vi "DVS_LabVIEWController_w_DAQ.vi"() -> ()   [LabVIEW 2013]
doc: "This example demonstrates temperature control and monitoring.\n\nNote:\nBefore start this VI is it necessary:\n\n- preconfigure some specific parameters that are not supported by this driver (e.g. PV-I/O Type, Linearization type, Alarm Input Values... ) by Quick Codes, or by Eurotherm iTools or by instrument front panel controls\n- enter correct VISA Resource Descriptor, Device Address and Baud Rate into front-panel controls"
uses:
  <vilib>/DAQmx/write.llb/DAQmx Write (Analog 1D DBL NChan 1Samp).vi
  <vilib>/DAQmx/read.llb/DAQmx Read (Analog 1D DBL NChan 1Samp).vi
  <vilib>/Utility/file.llb/Write To Spreadsheet File (string).vi
  <vilib>/Instr/_visa.llb/VISA Configure Serial Port (Instr).vi
  <vilib>/DAQmx/miscellaneous.llb/DAQmx Fill In Error Info.vi
  <instrlib>/Keithley 24XX/Public/Data/Read (Single Point).vi
  <instrlib>/Keithley 24XX/Keithley 24XX.lvlib
  <instrlib>/Eurotherm 32xx Series/Eurotherm 32xx Series.lvlib
panel:
  out "Waveform Chart 2":cluster{"f":dbl, "f":dbl}(graph)
  out "Waveform Chart 11":cluster{"Waveform":dbl, "Waveform":dbl}(graph)
  in  "Set vapor flow (sccm)":sgl min=0 max=200
  in  "Set gas flow (sccm)":sgl min=0 max=200
  out "Waveform Chart 10":dbl(graph)
  out "Vacuum Pressure (Torr)":dbl
  out "Waveform Chart 9":dbl(graph)
  out "Low pressure (Torr)":dbl
  out "Vapor flow (sccm)":dbl
  out "Gas flow (sccm)":dbl
  out "raw DVS DAQ data":dbl[](array[numeric])
  out "Waveform Chart 8":dbl(graph)
  out "High pressure (Torr)":dbl
  in  "Vacuum Data":bool
  in  "RapidOX":bool
  in  "Eurotherm Temp\nController":bool
  in  "4-wire?":bool
  in  "stop":bool
  in  "O2 PUMP":bool
  in  "QCM":bool
  in  "Keithley 2420":bool
  out "Data\nfile\npath":path
  in  "DATA COMMENTS":string
  out "ERRORS":errorcluster
  out "Starting time":string
  out "Elapsed (min)":dbl caption="Elapsed Time (s)"
  in  "Delay between data points (s)":dbl format="%#_13g"
  in  "Stop after (min)":dbl
  in  "Auto stop?":bool
  out "min remaining":dbl
  in  "Setpoint (C)":sgl=25.0
  out "Temp":T1(graph)
  out "Temp (C)":sgl
  in  "J-KEM":bool
  out "Freq (Hz)":dbl format="%.3e"
  out "R (Ohm)":dbl format="%.3e"
  out "Waveform Chart 7":T2(graph)
  out "Current Temp (C)":dbl
  in  "Setpoint (C)":dbl=25.0
  out "Current Setpoint (C)":dbl
  out "Waveform Chart 5":cluster{dbl, dbl}(graph)
  out "Waveform Chart":cluster{dbl}(graph)
  out "Torr":dbl
  out "%":dbl
  out "atm":dbl
  in  "Com Port":i32(ring) items=["Com 1", "Com 2", "Com 3", "Com 4", "Com 5", "Com 6", "COM 7", "COM 8", "COM 9", "COM 10", "COM 11", "COM 12", "com 13", "COM 14"]
  in  "Baud Rate 2":i32(ring)=2 items=["2400", "4800", "9600", "19200", "38400", "57600", "115200"]
  in  "Com Port 2":i32(ring) items=["Com 1", "Com 2", "Com 3", "Com 4", "Com 5", "Com 6", "COM 7", "COM 8", "COM 9", "COM 10", "COM 11", "COM 12", "com 13", "COM 14"]
  out "Waveform Chart 6":cluster{dbl}(graph)
  out "O2 Concentration (PPM)":dbl
  out "Resistance (Ohm)":sgl
  out "Waveform Chart 4":cluster{"Resistance":sgl}(graph)
  # "Keithley 2420\nRead Resistance"
  # "MKS Pressure Sensor"
  # "Configuring Instrument\n \nPlease Wait......\n\nChart will update in 20 sec"
  # "SRS QCM\nController"
  # "MKS Pressure Sensor"
  # "MKS Pressure Sensor"
  # "J-Kem Temp Control"
  # "O2 Partial Pressure"
  # "SetNag\nO2 Pump"
  # "Setup"
  # "Instruments Connected:"
  # "Timing"
  # "Eurotherm Temp Control"
  # "Rapidox O2\nSensor"
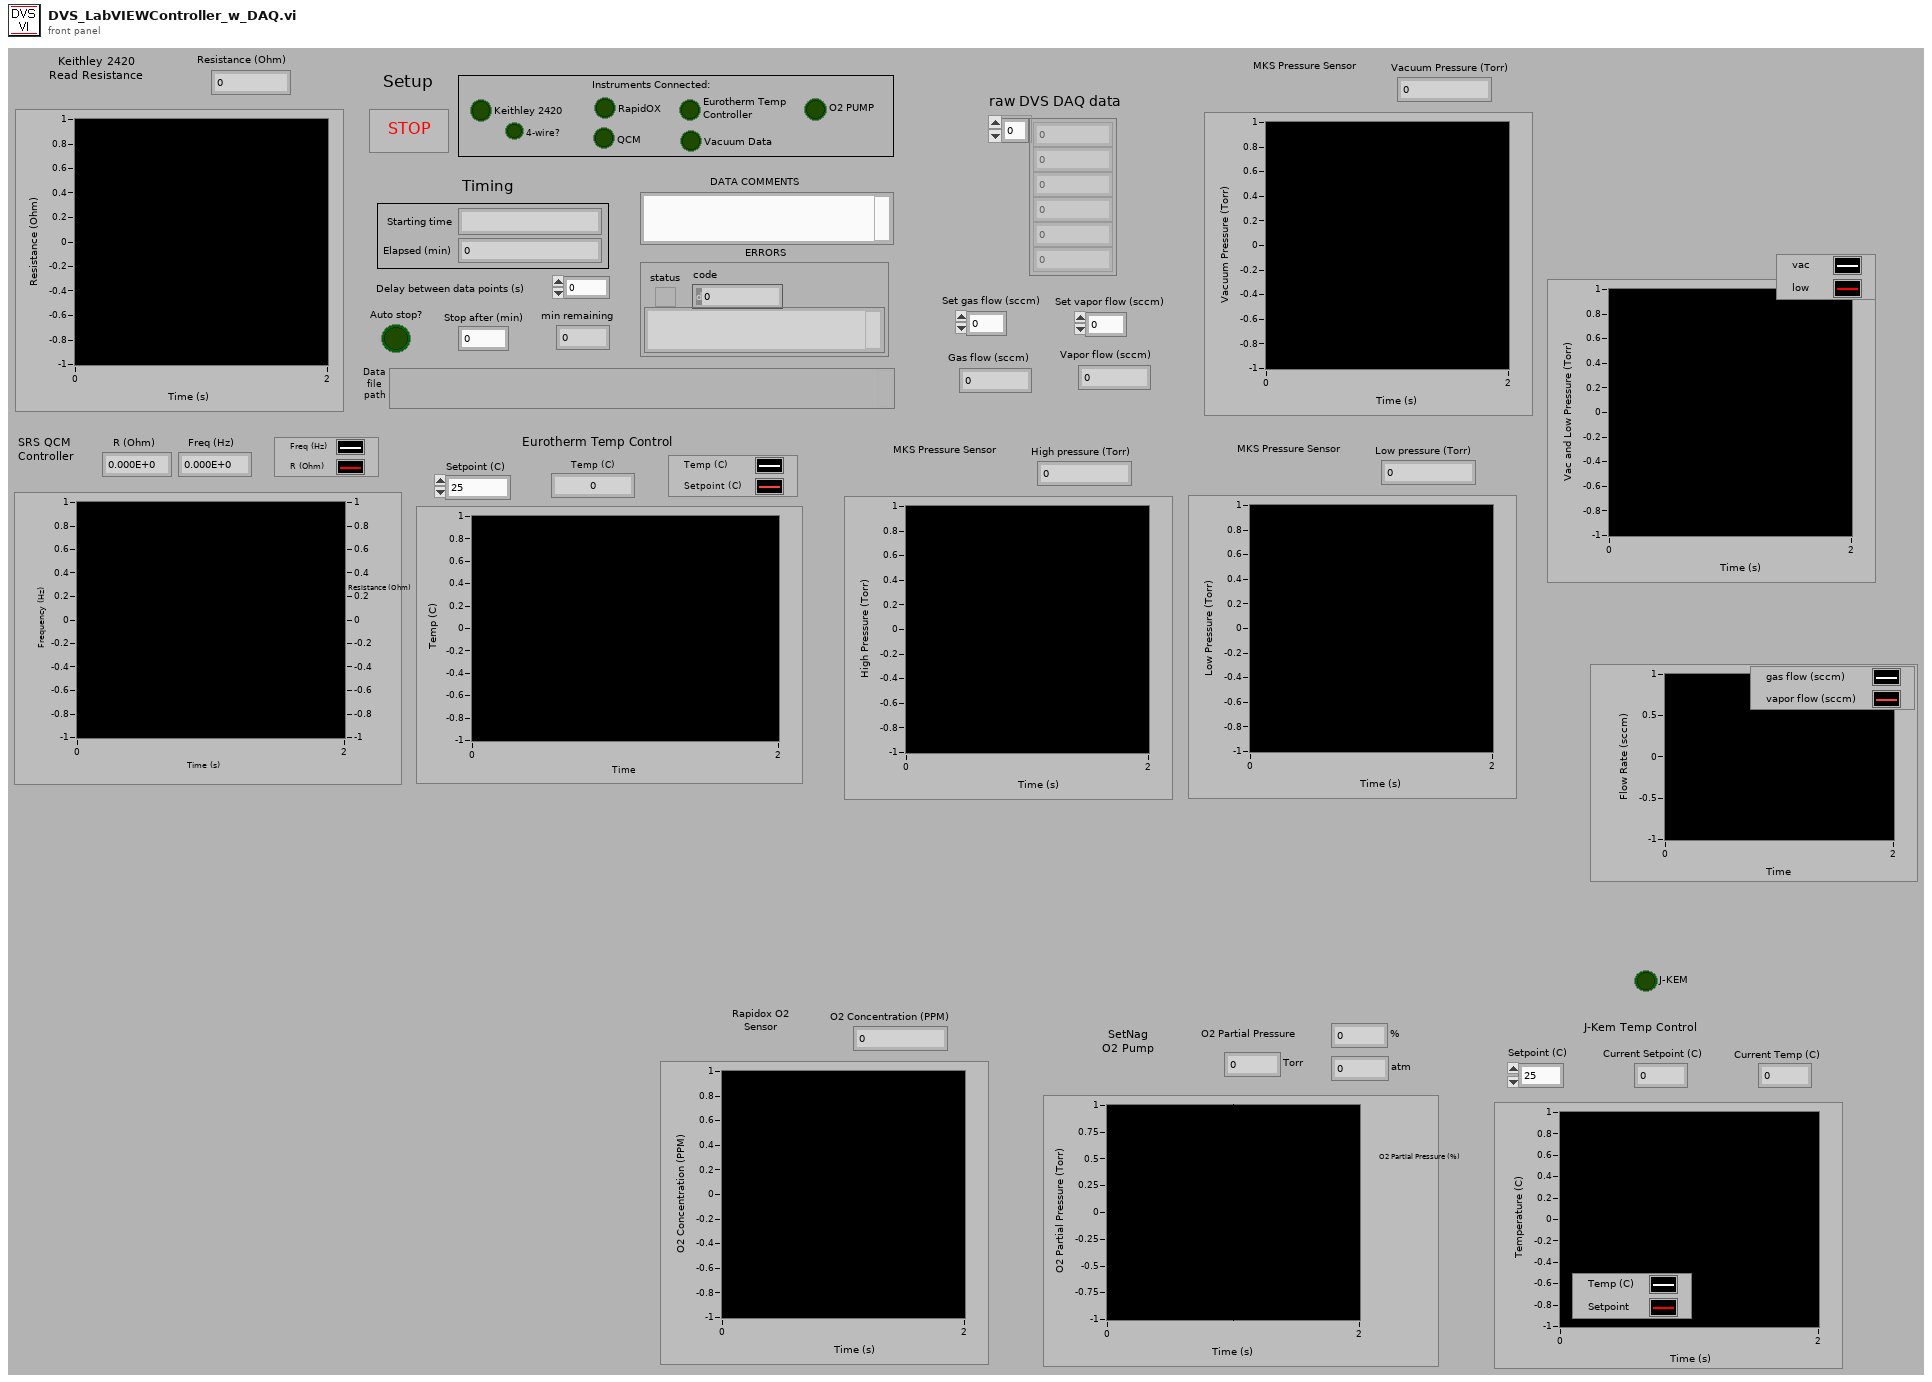
[diagram p1: front panel]
types:
  T1 = cluster{"Process Value":sgl, "Process Value":sgl}
  T2 = cluster{"Frequency out":dbl, "Resistance out":dbl}
  T3 = enum16{"open", "open or create", "create or replace", "create", "open (read only)"}
  T4 = cluster{bool, "Unit Address (1)":u8, "VISA resource name out":refnum<visa-resource-name>, "error out":errorcluster}
  T5 = cluster{"Process Value":sgl, "Setpoint Value 2":i16}[]
  T6 = cluster{"Baud Rate (19200)":u32, "Parity (0: None)":u16, "Break Length (0)":u16}
  T7 = enum16{"no parity", "odd parity", "even parity", "mark parity", "space parity"}
  T8 = cluster{bool, "VISA resource name":refnum<visa-resource-name>, "error out":errorcluster}
  T9 = cluster{bool, "VISA resource name out":refnum<visa-resource-name>, "error out":errorcluster}
  T10 = cluster{"Frequency out":dbl, "Resistance out":dbl}[]
  T11 = cluster{bool, "VISA out":refnum<visa-resource-name>, "error out":errorcluster}
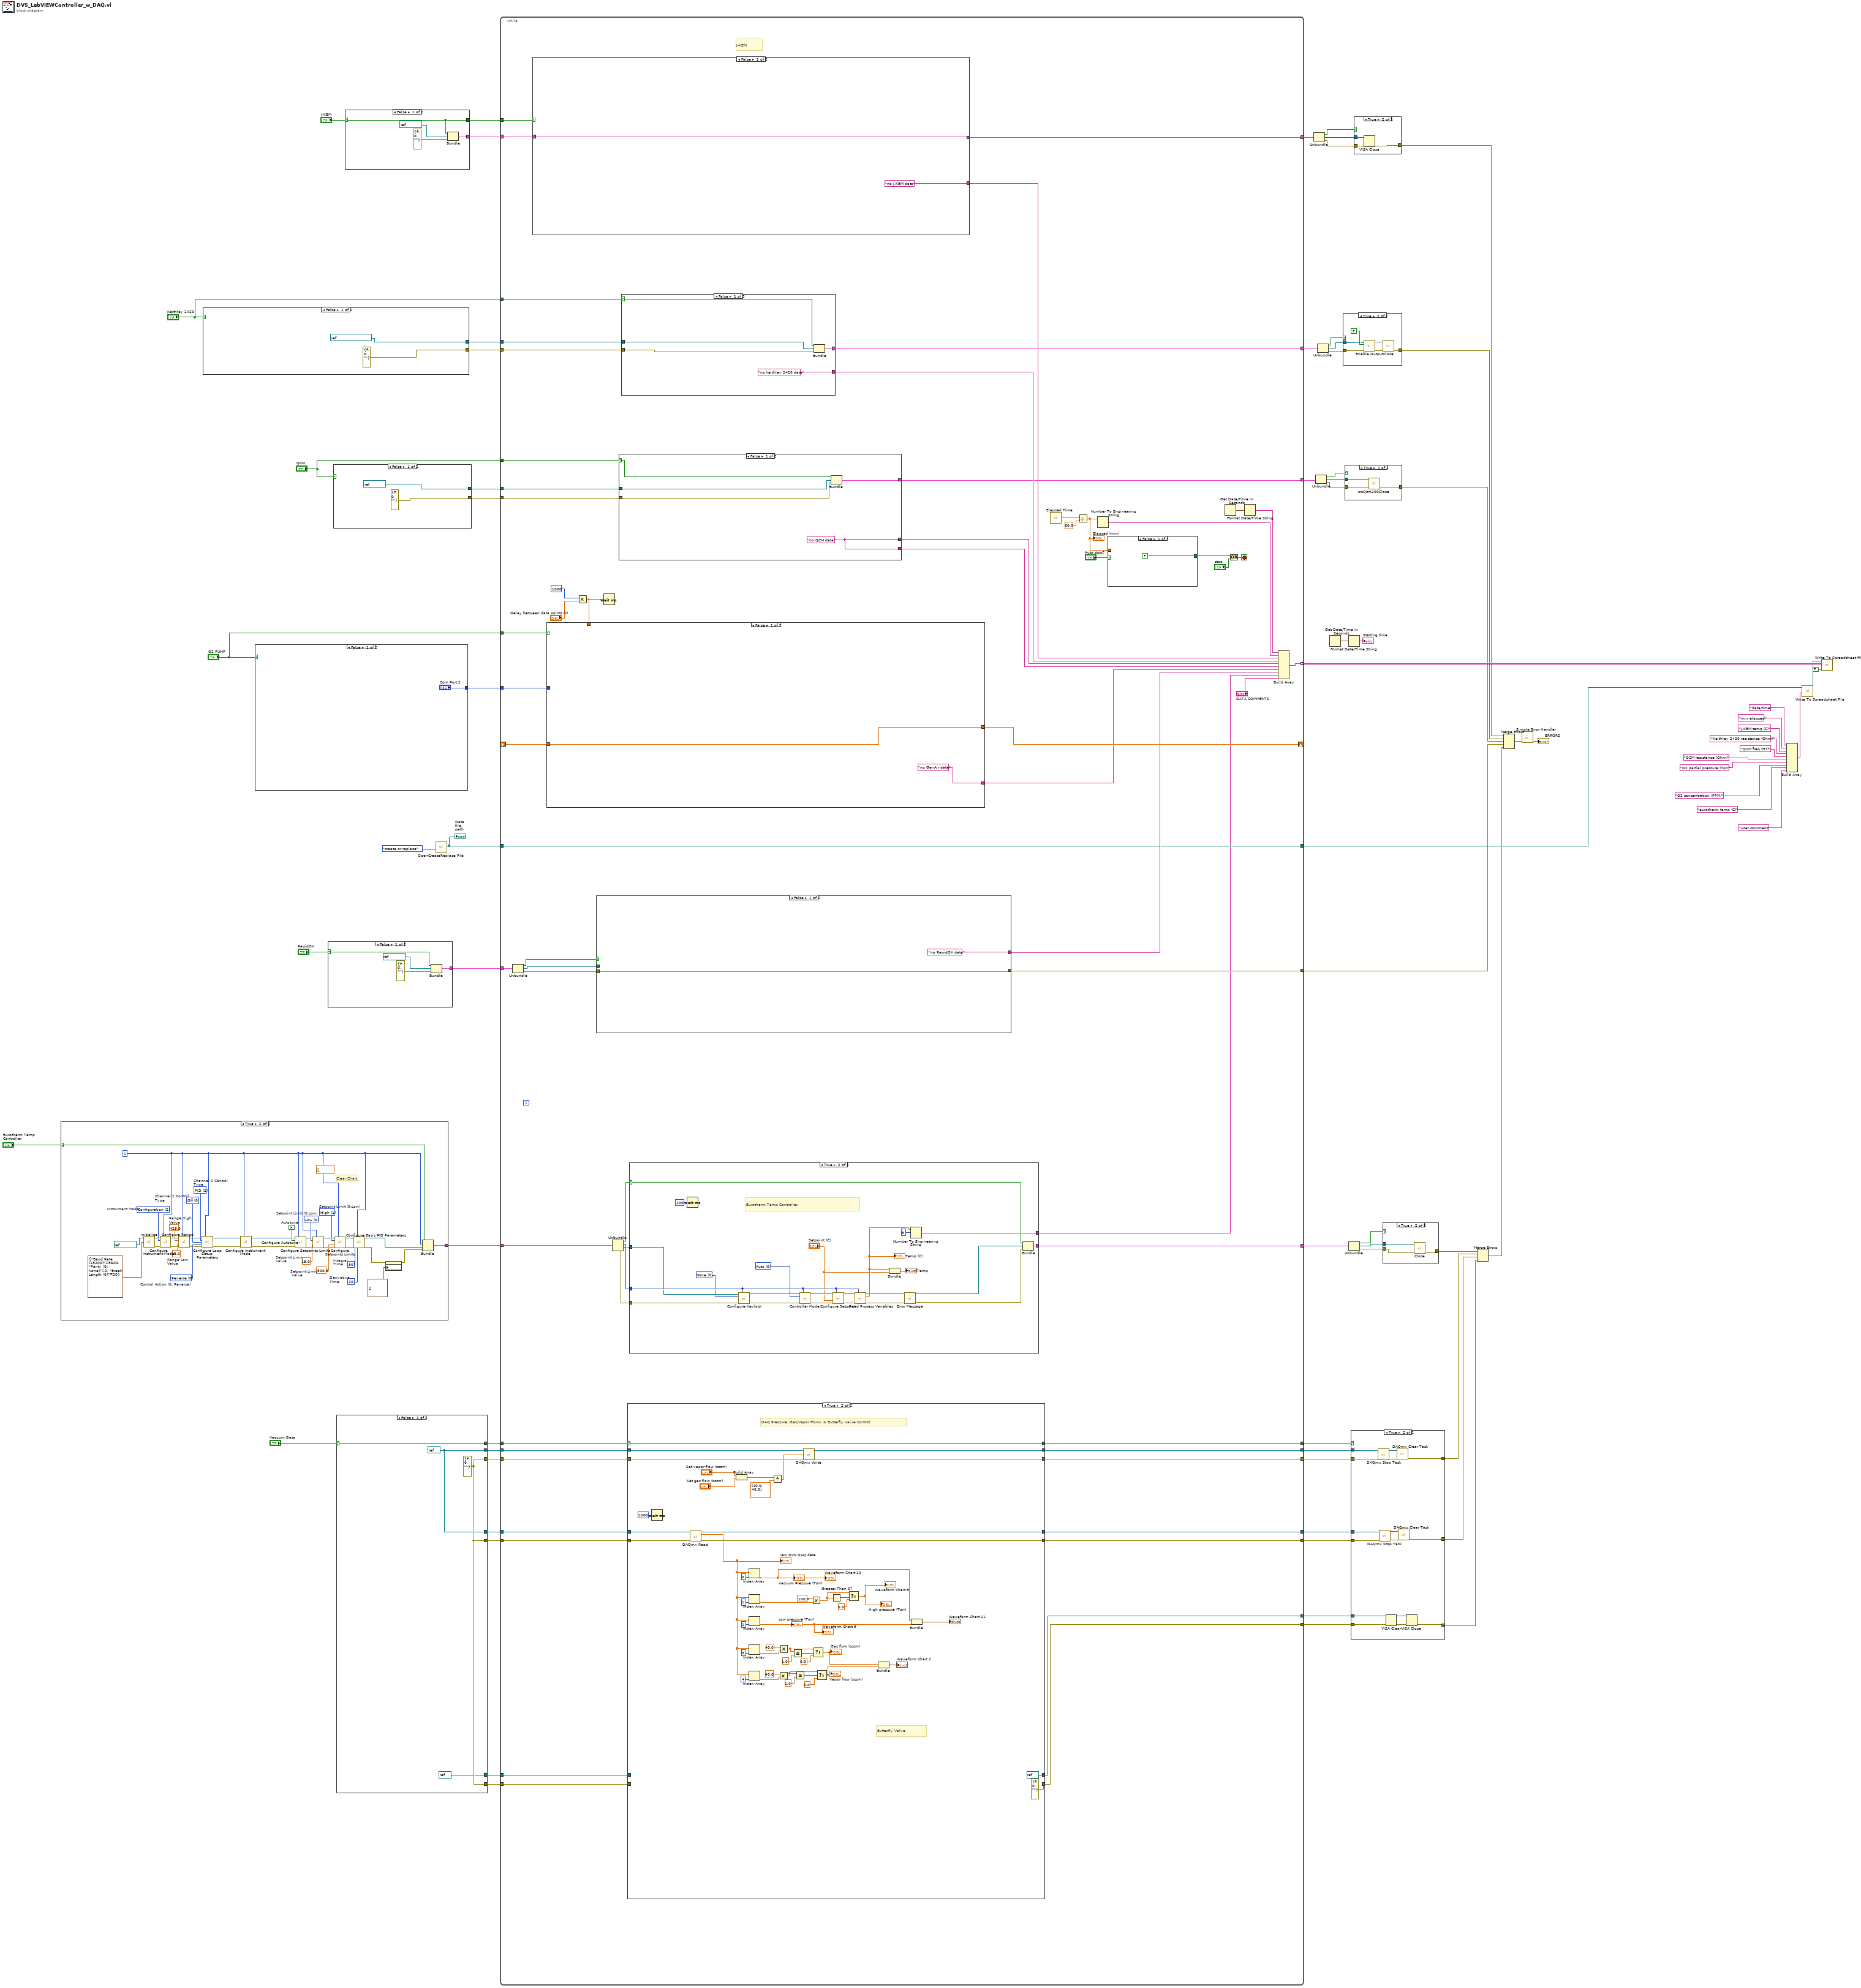
[diagram p0: block diagram]
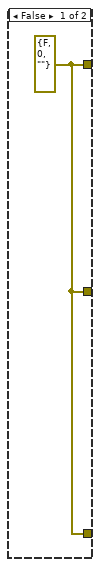
[diagram p2: hidden frame]
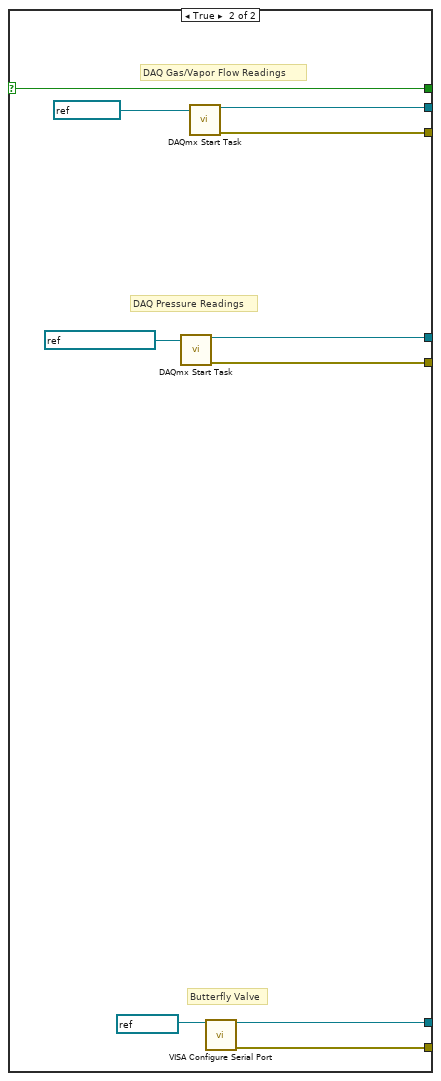
[diagram p3: hidden frame]
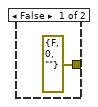
[diagram p4: hidden frame]
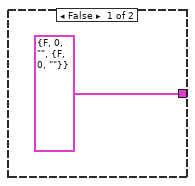
[diagram p5: hidden frame]
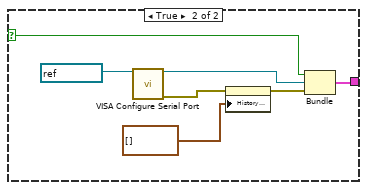
[diagram p6: hidden frame]
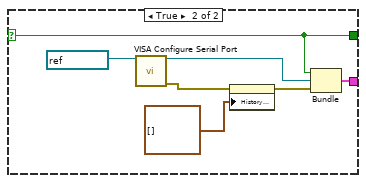
[diagram p8: hidden frame]
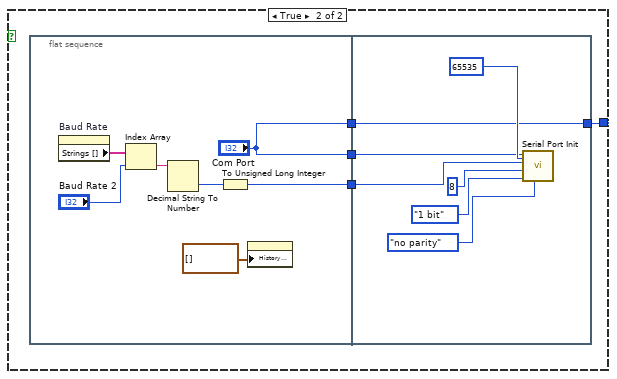
[diagram p9: hidden frame]
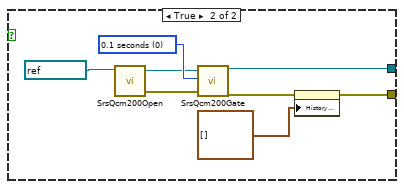
[diagram p11: hidden frame]
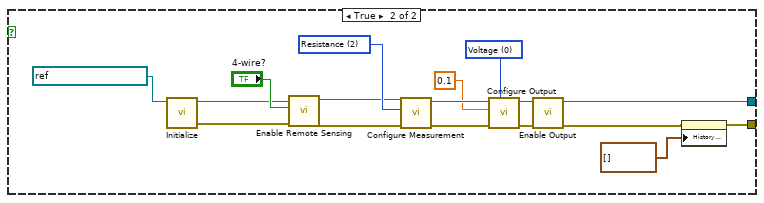
[diagram p13: hidden frame]
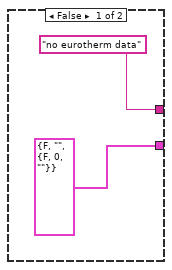
[diagram p15: hidden frame]
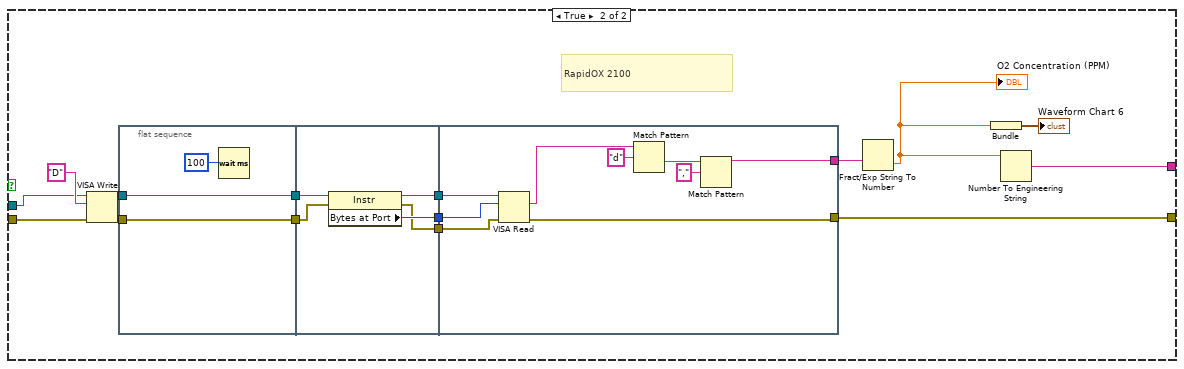
[diagram p16: hidden frame]
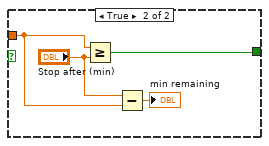
[diagram p17: hidden frame]
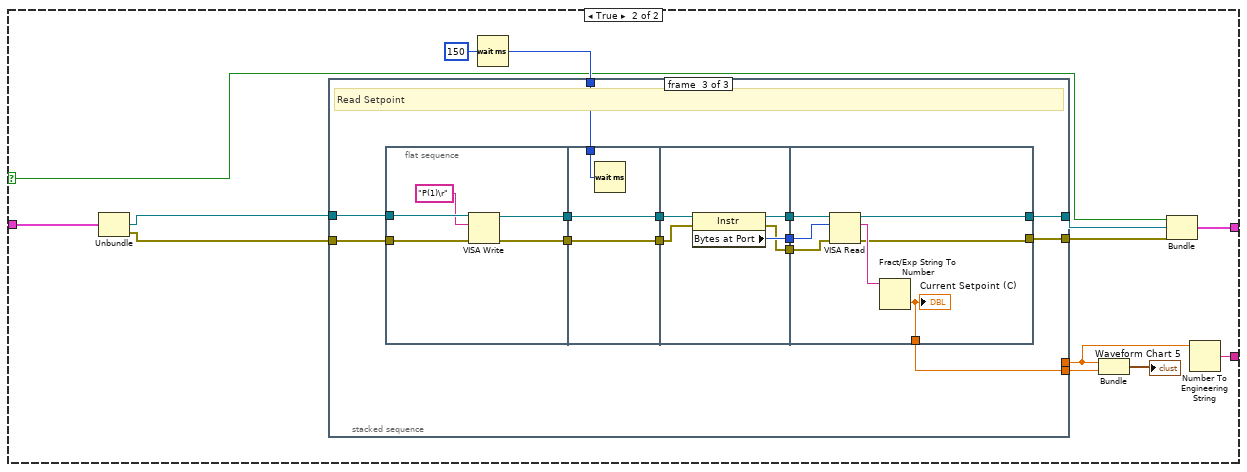
[diagram p18: hidden frame]
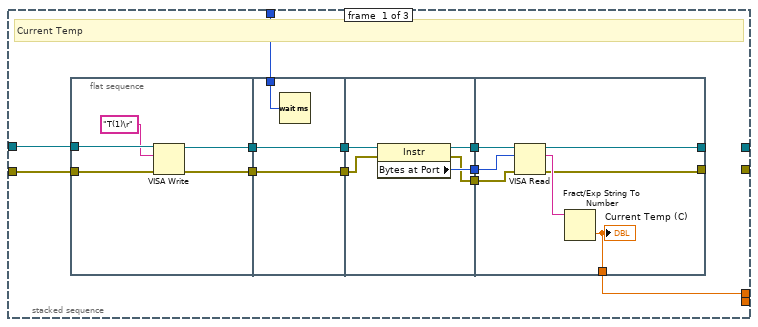
[diagram p19: hidden frame]
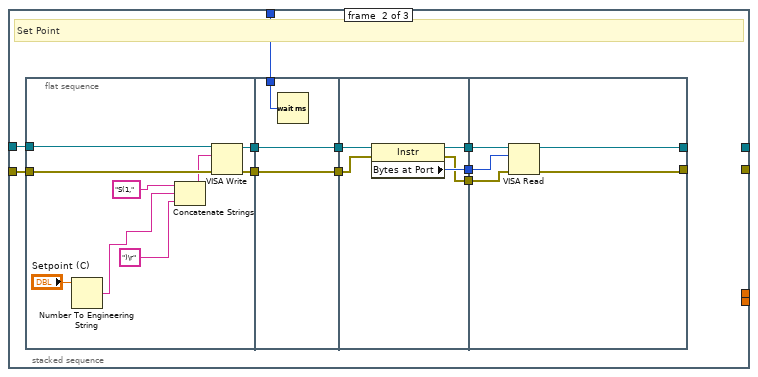
[diagram p20: hidden frame]
diagram:
  n1 = case shown="True" "Eurotherm Temp\nController" {
    selector: "Eurotherm Temp\nController" -> [_ w88]
    tunnel: [T4 {FALSE, "Unit Address (1)"=0, "VISA resource name out"="", "error out"={"status"=FALSE, "code"=0, "source"=""}} w85] -> w26
    frame False {
    }
    frame True {
      w87 = u8 1 ("Unit Address (1)")
      (unwired) sgl[] [] ("History Data")
      w92 = sgl 500.0  # Setpoint Limit  Value
      w95 = sgl 15.0  # Range Low  Value
      w96 = sgl 425.0  # Range High Value
      w97 = u16 0 items=["Reverse", "Direct"]  # Control Action (0: Reverse)
      w98 = u16 0 items=["Low", "High"]  # Setpoint Limit (0:Low)
      w99 = u16 1 items=["Low", "High"]  # Setpoint Limit (0:Low)
      w100 = 10  # Derivative  Time
      w101 = 50  # Integral  Time
      w102 = sgl 15.0  # Setpoint Limit  Value
      w107 = FALSE  # Autotune
      w110 = u8 0 items=["Off", "On/Off", "PID", "VPU", "VPB"]  # Channel 2 Control  Type
      w111 = u8 2 items=["Off", "On/Off", "PID", "VPU", "VPB"]  # Channel 1 Control  Type
      w114 = u8 2 items=["Normal", "StandBy", "Configuration"]  # Instrument Mode
      # "Clear Chart"
      n2 = call <instrlib>:"Initialize.vi"("VISA resource name"=refnum<visa-resource-name> "COM4", "Serial Configuration"=T6 {"Baud Rate (19200)"=9600, "Parity (0: None)"=0, "Break Length (0)"=20}) -> ("VISA resource name out"=w115:refnum<visa-resource-name>, "error out"=w91:errorcluster)  [unwired: 12 in]
      n3 = call <instrlib>:"Configure Instrument Mode.vi"("VISA resource name"=w115, "Unit Address (1)"=w87, "Instrument Mode (0: Normal)"=w114, "error in (no error)"=w91) -> ("VISA resource name out"=w113:refnum<visa-resource-name>, "error out"=w112:errorcluster)  [unwired: 10 in]
      n4 = call <instrlib>:"Configure Range.vi"("VISA resource name"=w113, "Unit Address (1)"=w87, "Range High (0)"=w96, "Range Low (0)"=w95, "error in (no error)"=w112) -> ("VISA resource name out"=w94:refnum<visa-resource-name>, "error out"=w93:errorcluster)  [unwired: 9 in]
      n5 = call <instrlib>:"Configure Loop Setup Parameters.vi"("VISA resource name"=w94, "Unit Address (1)"=w87, "Channel 1 Control Algorithm (0: Off)"=w111, "Channel 2 Control Algorithm (0: Off)"=w110, "Control Action (0: Reverse)"=w97, "error in (no error)"=w93) -> ("VISA resource name out"=w80:refnum<visa-resource-name>, "error out"=w81:errorcluster)  [unwired: 8 in]
      n6 = call <instrlib>:"Configure Instrument Mode.vi"("VISA resource name"=w80, "Unit Address (1)"=w87, "error in (no error)"=w81) -> ("VISA resource name out"=w79:refnum<visa-resource-name>, "error out"=w78:errorcluster)  [unwired: 11 in]
      n7 = call <instrlib>:"Configure Autotune.vi"("VISA resource name"=w79, "Unit Address (1)"=w87, "Enable Autotune  (False: Disable)"=w107, "error in (no error)"=w78) -> ("VISA resource name out"=w106:refnum<visa-resource-name>, "error out"=w105:errorcluster)  [unwired: 10 in]
      n8 = call <instrlib>:"Configure Setpoints Limits.vi"("VISA resource name"=w106, "Unit Address (1)"=w87, "Setpoint Limit (0:Low)"=w98, "Setpoint Limit Value (0)"=w102, "error in (no error)"=w105) -> ("VISA resource name out"=w109:refnum<visa-resource-name>, "error out"=w108:errorcluster)  [unwired: 9 in]
      n9 = call <instrlib>:"Configure Setpoints Limits.vi"("VISA resource name"=w109, "Unit Address (1)"=w87, "Setpoint Limit (0:Low)"=w99, "Setpoint Limit Value (0)"=w92, "error in (no error)"=w108) -> ("VISA resource name out"=w104:refnum<visa-resource-name>, "error out"=w103:errorcluster)  [unwired: 9 in]
      n10 = call <instrlib>:"Configure Basic PID Parameters.vi"("VISA resource name"=w104, "Unit Address (1)"=w87, "Integral Time (1)"=w101, "error in (no error)"=w103, "Derivative Time (0)"=w100) -> ("VISA resource name out"=w86:refnum<visa-resource-name>, "error out"=w83:errorcluster)  [unwired: 9 in]
      n11 = property on="Temp" class="WFChart (strict)"(error in=w83, "History Data"=T5 []) -> (error out=w82:errorcluster)  [unwired: 1 in, 1 out]
      n12 = Bundle(w88, "Unit Address (1)"=w87, "VISA resource name out"=w86, "error out"=w82) -> (w85:T4)  [unwired: 1 in]
    }
  }
  n13 = case shown="False" "Keithley 2420" {
    tunnel: [refnum<visa-resource-name> "GPIB1::24::INSTR" ("VISA resource name") w122] -> w70
    tunnel: [errorcluster {"status"=FALSE, "code"=0, "source"=""} ("error out") w125] -> w69
    frame False {
    }
    frame True {
      w128 = u16 0 items=["Voltage", "Current"] ("Source Mode  (0: Voltage)")
      w133 = u16 2 items=["Volts", "Current", "Resistance"] ("Function (0: Volts)")
      n14 = call <instrlib>:"Initialize.vi"("VISA resource name"=refnum<visa-resource-name> "GPIB1::24::INSTR") -> ("error out"=w118:errorcluster, "VISA resource name out"=w121:refnum<visa-resource-name>)  [unwired: 9 in]
      n15 = call <instrlib>:"Enable Remote Sensing.vi"("error in (no error)"=w118, "Enable Remote Sensing (T: Enable)"="4-wire?", "VISA resource name"=w121) -> ("error out"=w119:errorcluster, "VISA resource name out"=w120:refnum<visa-resource-name>)  [unwired: 7 in]
      n16 = call <instrlib>:"Configure Measurement.vi"("error in (no error)"=w119, "Function (0: Volts)"=w133, "VISA resource name"=w120) -> ("error out"=w132:errorcluster, "VISA resource name out"=w131:refnum<visa-resource-name>)  [unwired: 7 in]
      n17 = call <instrlib>:"Configure Output.vi"("Source Mode  (0: Voltage)"=w128, "error in (no error)"=w132, "Output Level (0)"=0.1 ("Output Level (V)"), "VISA resource name"=w131) -> ("error out"=w130:errorcluster, "VISA resource name out"=w129:refnum<visa-resource-name>)  [unwired: 6 in]
      n18 = call <instrlib>:"Enable Output.vi"("error in (no error)"=w130, "VISA resource name"=w129) -> ("error out"=w123:errorcluster, "VISA resource name out"=w122:refnum<visa-resource-name>)  [unwired: 8 in]
      n19 = property on="Waveform Chart 4" class="WFChart (strict)"(error in=w123, "History Data"=cluster{"Resistance":sgl}[] []) -> (error out=w125:errorcluster)  [unwired: 1 in, 1 out]
    }
  }
  n20 = case shown="False" "O2 PUMP" {
    tunnel: ["Com Port 2" w136] -> w64
    frame False {
    }
    frame True {
      n21 = flat-sequence {
        tunnel: ["Com Port"] -> w139
        tunnel: [w142] -> w138
        tunnel: ["Com Port"] -> w137
        tunnel: w139 -> [w148]
        tunnel: w138 -> [w147]
        tunnel: w137 -> [w149]
        tunnel: [w149] -> w136
        frame #0 {
          n22 = property on="Baud Rate" class="Ring (strict)"() -> ("Strings []"=w144:string[])  [unwired: 2 in, 2 out]
          n23 = Index Array(array=w144, index="Baud Rate 2") -> (element=w145:string)
          n24 = Decimal String To Number(string=w145) -> (number=w143:i32)  [unwired: 2 in, 1 out]
          n25 = To Unsigned Long Integer(number=w143) -> (unsigned 32bit integer=w142:u32)
          n26 = property on="Waveform Chart" class="WFChart (strict)"("History Data"=cluster{dbl}[] []) -> ()  [unwired: 2 in, 2 out]
        }
        frame #1 {
          n27 = call <vilib>:"Serial Port Init.vi"("parity"=T7."no parity", "buffer size"=u16 65535, "stop bits"=enum16{"1 bit", "1.5 bits", "2 bits"}."1 bit", "data bits"=u16 8, "baud rate"=w147, "port number"=w148) -> ()  [unwired: 1 in, 1 out]
        }
      }
    }
  }
  n28 = case shown="False" "RapidOX" {
    selector: "RapidOX" -> [w154 w161]
    tunnel: [w155 w162] -> w32
    frame False {
      n29 = Bundle(w154, "VISA resource name"=refnum<visa-resource-name> "COM7", "error out"=errorcluster {"status"=FALSE, "code"=0, "source"=""}) -> (w155:T8)  [unwired: 1 in]
    }
    frame True {
      n30 = call-poly "VISA Configure Serial Port"("VISA resource name"=refnum<visa-resource-name> "COM7") -> ("VISA resource name out"=w163:refnum<visa-resource-name>, "error out"=w159:errorcluster)  [unwired: 13 in]
      n31 = property on="Waveform Chart 6" class="WFChart (strict)"(error in=w159, "History Data"=cluster{dbl}[] []) -> (error out=w158:errorcluster)  [unwired: 1 in, 1 out]
      n32 = Bundle(w161, "VISA resource name out"=w163, "error out"=w158) -> (w162:T9)  [unwired: 1 in]
    }
  }
  n33 = case shown="False" "QCM" {
    tunnel: [refnum<visa-resource-name> "COM6" ("VISA in") w170] -> w68
    tunnel: [errorcluster {"status"=FALSE, "code"=0, "source"=""} ("error out") w168] -> w67
    frame False {
    }
    frame True {
      w174 = u16 0 items=["0.1 seconds", "1.0 seconds", "10.0 seconds"] ("Gate in")
      n34 = call <instrlib>:"SrsQcm200Open.vi"("VISA in"=refnum<visa-resource-name> "COM6") -> ("error out"=w171:errorcluster, "VISA out"=w172:refnum<visa-resource-name>)  [unwired: 4 in]
      n35 = call <instrlib>:"SrsQcm200Gate.vi"("VISA in"=w172, "Gate in"=w174, "error in (no error)"=w171) -> ("VISA out"=w170:refnum<visa-resource-name>, "error out"=w167:errorcluster)  [unwired: 14 in, 1 out]
      n36 = property on="Waveform Chart 7" class="WFChart (strict)"(error in=w167, "History Data"=T10 []) -> (error out=w168:errorcluster)  [unwired: 1 in, 1 out]
    }
  }
  n37 = case shown="False" "Vacuum Data" {
    selector: "Vacuum Data" -> [w178 w186]
    tunnel: [w177 w187] -> w19
    tunnel: [w178 w186] -> w18
    tunnel: [w176 w185] -> w17
    tunnel: [w177 w183] -> w11
    tunnel: [w176 w182] -> w10
    tunnel: [refnum<visa-resource-name> refnum ("VISA resource name out") w179] -> w5
    tunnel: [w176 w180] -> w4
    frame False {
      w176 = errorcluster {"status"=FALSE, "code"=0, "source"=""} ("error out")
      w177 = refnum<k21> refnum ("task out")
    }
    frame True {
      # "DAQ Gas/Vapor Flow Readings"
      # "DAQ Pressure Readings"
      # "Butterfly Valve"
      n38 = call <vilib>:"DAQmx Start Task.vi"("task/channels in"=refnum<k21> "AllDaqReadings") -> ("task out"=w187:refnum<k21>, "error out"=w185:errorcluster)  [unwired: 13 in]
      n39 = call <vilib>:"DAQmx Start Task.vi"("task/channels in"=refnum<k21> "Setflow") -> ("task out"=w183:refnum<k21>, "error out"=w182:errorcluster)  [unwired: 13 in]
      n40 = call-poly "VISA Configure Serial Port"("VISA resource name"=refnum<visa-resource-name> "COM5") -> ("VISA resource name out"=w179:refnum<visa-resource-name>, "error out"=w180:errorcluster)  [unwired: 13 in]
    }
  }
  n41 = case shown="False" "J-KEM" {
    selector: "J-KEM" -> [w189 w196]
    tunnel: [w190 w197] -> w53
    tunnel: [w189 w196] -> w46
    frame False {
      n42 = Bundle(w189, "VISA resource name"=refnum<visa-resource-name> "COM3", "error out"=errorcluster {"status"=FALSE, "code"=0, "source"=""}) -> (w190:T8)  [unwired: 1 in]
    }
    frame True {
      n43 = call-poly "VISA Configure Serial Port"("VISA resource name"=refnum<visa-resource-name> "COM3") -> ("VISA resource name out"=w198:refnum<visa-resource-name>, "error out"=w194:errorcluster)  [unwired: 13 in]
      n44 = property on="Waveform Chart 5" class="WFChart (strict)"(error in=w194, "History Data"=cluster{dbl, dbl}[] []) -> (error out=w193:errorcluster)  [unwired: 1 in, 1 out]
      n45 = Bundle(w196, "VISA resource name out"=w198, "error out"=w193) -> (w197:T9)  [unwired: 1 in]
    }
  }
  n46 = call <instrlib>:"OpenCreateReplace File.vi"("function (open:0)"=T3."create or replace") -> ("new file path"=w28:path)  [unwired: 7 in, 3 out]
  "Data\nfile\npath" <- w28
  n47 = while {
    shift-right: [w260] -> _
    shift-left: _ -> [w259]
    tunnel: [w257] -> w72 mode=indexing
    tunnel: "Keithley 2420" -> [w223]
    tunnel: w70 -> [w255]
    tunnel: w69 -> [w254]
    tunnel: w68 -> [w253]
    tunnel: w67 -> [w252]
    tunnel: "QCM" -> [w250]
    tunnel: "O2 PUMP" -> [w243]
    tunnel: w64 -> [w249]
    tunnel: [w245] -> w61
    tunnel: [w244] -> w57
    tunnel: w53 -> [w242]
    tunnel: [w241] -> w51
    tunnel: w46 -> [w239]
    tunnel: w32 -> [w232]
    tunnel: [w227] -> w30
    tunnel: [w221] -> w29
    tunnel: w28 -> [w221]
    tunnel: w26 -> [w220]
    tunnel: [w218] -> w25
    tunnel: w19 -> [w213]
    tunnel: w18 -> [w212]
    tunnel: w17 -> [w211]
    tunnel: [w210] -> w16
    tunnel: [w209] -> w15
    tunnel: [w208] -> w14
    tunnel: w11 -> [w207]
    tunnel: w10 -> [w206]
    tunnel: [w205] -> w9
    tunnel: [w204] -> w8
    tunnel: w5 -> [w203]
    tunnel: w4 -> [w201]
    tunnel: [w202] -> w3
    tunnel: [w200] -> w2
    stop <- w237 stop-if-true
    # "J-KEM"
    n48 = Unbundle(w232) -> (w231:bool, "VISA resource name out"=w230:refnum<visa-resource-name>, "error out"=w229:errorcluster)
    n49 = case shown="False" w239 {
      selector: w239 -> [_ w384]
      tunnel: w242 -> [w382 w389]
      tunnel: [w382 w387] -> w241
      tunnel: ["no J-KEM data" w385] -> w240
      frame False {
      }
      frame True {
        w394 = u32 150 ("milliseconds to wait")
        n50 = Unbundle(w389) -> ("VISA resource name out"=w388:refnum<visa-resource-name>, "error out"=w383:errorcluster)  [unwired: 1 out]
        n51 = stacked-sequence {
          tunnel: w388 -> [w398 w428 w462]
          tunnel: w383 -> [w397 w427 w461]
          tunnel: w394 -> [w396 w426 w463]
          tunnel: [_ _ w460] -> w390
          tunnel: [_ _ w459] -> w391
          tunnel: [w395 _ _] -> w386
          tunnel: [_ _ w458] -> w393
          frame #0 {
            # "Current Temp"
            n52 = flat-sequence {
              tunnel: w398 -> [w410]
              tunnel: w397 -> [w409]
              tunnel: [w407] -> w405
              tunnel: [w406] -> w404
              tunnel: w396 -> [w413]
              tunnel: [w412] -> w403
              tunnel: w405 -> [w412]
              tunnel: w404 -> [w411]
              tunnel: [w411] -> w402
              tunnel: w403 -> [w418]
              tunnel: w402 -> [w417]
              tunnel: [w416] -> w401
              tunnel: [w415] -> w400
              tunnel: [w414] -> w399
              tunnel: w401 -> [w425]
              tunnel: w400 -> [w424]
              tunnel: w399 -> [w423]
              tunnel: [w420] -> _
              tunnel: [w421] -> _
              tunnel: [w419] -> w395
              frame #0 {
                n53 = VISA Write(VISA resource name=w410, write buffer="T(1)\r", error in (no error)=w409) -> (VISA resource name out=w407:refnum<visa-resource-name>, error out=w406:errorcluster)  [unwired: 1 out]
              }
              frame #1 {
                n54 = Wait (ms)(milliseconds to wait=w413) -> ()  [unwired: 1 out]
              }
              frame #2 {
                n55 = property class="Instr"(reference=w418, error in=w417) -> (reference out=w416:refnum<visa-resource-name>, error out=w414:errorcluster, "Bytes at Port"=w415:u32)
              }
              frame #3 {
                n56 = VISA Read(VISA resource name=w425, byte count=w424, error in (no error)=w423) -> (VISA resource name out=w421:refnum<visa-resource-name>, read buffer=w422:string, error out=w420:errorcluster)  [unwired: 1 out]
                n57 = Fract/Exp String To Number(string=w422) -> (number=w419:dbl)  [unwired: 3 in, 1 out]
                "Current Temp (C)" <- w419
              }
            }
          }
          frame #1 {
            # "Set Point"
            n58 = flat-sequence {
              tunnel: w428 -> [w444]
              tunnel: w427 -> [w443]
              tunnel: [w442] -> w435
              tunnel: [w441] -> w434
              tunnel: w426 -> [w447]
              tunnel: [w446] -> w433
              tunnel: w435 -> [w446]
              tunnel: w434 -> [w445]
              tunnel: [w445] -> w432
              tunnel: w433 -> [w452]
              tunnel: w432 -> [w451]
              tunnel: [w450] -> w431
              tunnel: [w449] -> w430
              tunnel: [w448] -> w429
              tunnel: w431 -> [w457]
              tunnel: w430 -> [w456]
              tunnel: w429 -> [w455]
              tunnel: [w453] -> _
              tunnel: [w454] -> _
              frame #0 {
                n59 = Number To Engineering String(4:"Setpoint (C)") -> (0:w437:string)  [unwired: 3 in]
                n60 = Concatenate Strings("S(1," ("write buffer"), w437, ")\r" ("write buffer")) -> (w440:string)
                n61 = VISA Write(VISA resource name=w444, write buffer=w440, error in (no error)=w443) -> (VISA resource name out=w442:refnum<visa-resource-name>, error out=w441:errorcluster)  [unwired: 1 out]
              }
              frame #1 {
                n62 = Wait (ms)(milliseconds to wait=w447) -> ()  [unwired: 1 out]
              }
              frame #2 {
                n63 = property class="Instr"(reference=w452, error in=w451) -> (reference out=w450:refnum<visa-resource-name>, error out=w448:errorcluster, "Bytes at Port"=w449:u32)
              }
              frame #3 {
                n64 = VISA Read(VISA resource name=w457, byte count=w456, error in (no error)=w455) -> (VISA resource name out=w454:refnum<visa-resource-name>, error out=w453:errorcluster)  [unwired: 2 out]
              }
            }
          }
          frame #2 {
            # "Read Setpoint"
            n65 = flat-sequence {
              tunnel: w462 -> [w475]
              tunnel: w461 -> [w474]
              tunnel: [w472] -> w470
              tunnel: [w471] -> w469
              tunnel: [w478] -> w468
              tunnel: w470 -> [w478]
              tunnel: w469 -> [w477]
              tunnel: [w477] -> w467
              tunnel: w463 -> [w476]
              tunnel: w468 -> [w483]
              tunnel: w467 -> [w482]
              tunnel: [w481] -> w466
              tunnel: [w480] -> w465
              tunnel: [w479] -> w464
              tunnel: w466 -> [w490]
              tunnel: w465 -> [w489]
              tunnel: w464 -> [w488]
              tunnel: [w485] -> w459
              tunnel: [w486] -> w460
              tunnel: [w484] -> w458
              frame #0 {
                n66 = VISA Write(VISA resource name=w475, write buffer="P(1)\r", error in (no error)=w474) -> (VISA resource name out=w472:refnum<visa-resource-name>, error out=w471:errorcluster)  [unwired: 1 out]
              }
              frame #1 {
                n67 = Wait (ms)(milliseconds to wait=w476) -> ()  [unwired: 1 out]
              }
              frame #2 {
                n68 = property class="Instr"(reference=w483, error in=w482) -> (reference out=w481:refnum<visa-resource-name>, error out=w479:errorcluster, "Bytes at Port"=w480:u32)
              }
              frame #3 {
                n69 = VISA Read(VISA resource name=w490, byte count=w489, error in (no error)=w488) -> (VISA resource name out=w486:refnum<visa-resource-name>, read buffer=w487:string, error out=w485:errorcluster)  [unwired: 1 out]
                n70 = Fract/Exp String To Number(string=w487) -> (number=w484:dbl)  [unwired: 3 in, 1 out]
                "Current Setpoint (C)" <- w484
              }
            }
          }
        }
        n71 = Wait (ms)(milliseconds to wait=w394) -> ()  [unwired: 1 out]
        n72 = Bundle(w386, w393) -> (→"Waveform Chart 5":cluster{dbl, dbl})  [unwired: 1 in]
        n73 = Bundle(w384, "VISA resource name out"=w390, "error out"=w391) -> (w387:T9)  [unwired: 1 in]
        n74 = Number To Engineering String(4:w386) -> (0:w385:string)  [unwired: 3 in]
      }
    }
    n75 = Multiply(x=u32 1000, y="Delay between data points (s)") -> (x*y=w226:dbl)
    n76 = case shown="False" w243 {
      tunnel: [w525 w529] -> w260
      tunnel: w259 -> [w525 w530]
      tunnel: w226 -> [_ w526]
      tunnel: w249 -> [_ w528]
      tunnel: ["no GenAir data" w527] -> w248
      frame False {
      }
      frame True {
        # "SetNag O2 Gauge"
        n77 = flat-sequence {
          tunnel: [w539] -> w536
          tunnel: w526 -> [w541]
          tunnel: w528 -> [w539]
          tunnel: w536 -> [w542]
          tunnel: w526 -> [w549]
          tunnel: [w545] -> w529
          frame #0 {
            n78 = Wait (ms)(milliseconds to wait=w541) -> ()  [unwired: 1 out]
            n79 = call <vilib>:"Serial Port Write.vi"("string to write"="_OXY\r" ("O2 partial press"), "port number"=w539) -> ()  [unwired: 1 out]
          }
          frame #1 {
            # "O2 partial pressure"
            n80 = call <vilib>:"Bytes At Serial Port.vi"() -> ("byte count"=w550:u32)  [unwired: 1 in, 1 out]
            n81 = Wait (ms)(milliseconds to wait=w549) -> ()  [unwired: 1 out]
            n82 = call <vilib>:"Serial Port Read.vi"("requested byte count"=w550, "port number"=w542) -> ("string read"=w548:string)  [unwired: 1 out]
            n83 = Fract/Exp String To Number(string=w548) -> (number=w546:dbl)  [unwired: 3 in, 1 out]
            "atm" <- w546
            n84 = Multiply(x=w546, y=100.0) -> (x*y=w543:dbl)
            "%" <- w543
            n85 = Multiply(x=w543, y=7.6) -> (x*y=w545:dbl)
            "Torr" <- w545
          }
        }
        n86 = Wait (ms)(milliseconds to wait=w526) -> ()  [unwired: 1 out]
        n87 = Greater?(x=w529, y=1e-07) -> (0:w532:bool)
        n88 = case shown="False" w532 {
          tunnel: [w537 w538] -> w531
          tunnel: w529 -> [_ w538]
          tunnel: w530 -> [w537 _]
          frame False {
          }
          frame True {
          }
        }
        n89 = Number To Engineering String(4:w531) -> (0:w527:string)  [unwired: 3 in]
        n90 = Bundle(w527) -> (w534:cluster{string})  [unwired: 1 in]
        n91 = Fract/Exp String To Number(string=w534) -> (number=→"Waveform Chart":cluster{dbl})  [unwired: 3 in, 1 out]
      }
    }
    n92 = case shown="False" w231 {
      tunnel: w230 -> [_ w349]
      tunnel: w229 -> [w342 w348]
      tunnel: ["no RapidOX data" w347] -> w228
      tunnel: [w342 w344] -> w227
      frame False {
      }
      frame True {
        # "RapidOX 2100"
        n93 = VISA Write(VISA resource name=w349, write buffer="D", error in (no error)=w348) -> (VISA resource name out=w352:refnum<visa-resource-name>, error out=w351:errorcluster)  [unwired: 1 out]
        n94 = flat-sequence {
          tunnel: [w361] -> w358
          tunnel: [w359] -> w357
          tunnel: w352 -> [w361]
          tunnel: w351 -> [w359]
          tunnel: w358 -> [w366]
          tunnel: w357 -> [w365]
          tunnel: [w364] -> w356
          tunnel: [w363] -> w355
          tunnel: [w362] -> w354
          tunnel: w356 -> [w375]
          tunnel: w355 -> [w374]
          tunnel: w354 -> [w373]
          tunnel: [w372] -> w344
          tunnel: [w367] -> w346
          frame #0 {
            n95 = Wait (ms)(milliseconds to wait=u32 100) -> ()  [unwired: 1 out]
          }
          frame #1 {
            n96 = property class="Instr"(reference=w366, error in=w365) -> (reference out=w364:refnum<visa-resource-name>, error out=w362:errorcluster, "Bytes at Port"=w363:u32)
          }
          frame #2 {
            n97 = VISA Read(VISA resource name=w375, byte count=w374, error in (no error)=w373) -> (read buffer=w370:string, error out=w372:errorcluster)  [unwired: 2 out]
            n98 = Match Pattern(string=w370, regular expression="d") -> (after substring=w368:string)  [unwired: 1 in, 3 out]
            n99 = Match Pattern(string=w368, regular expression=",") -> (before substring=w367:string)  [unwired: 1 in, 3 out]
          }
        }
        n100 = Fract/Exp String To Number(string=w346) -> (number=w345:dbl)  [unwired: 3 in, 1 out]
        "O2 Concentration (PPM)" <- w345
        n101 = Bundle(w345) -> (→"Waveform Chart 6":cluster{dbl})  [unwired: 1 in]
        n102 = Number To Engineering String(4:w345) -> (0:w347:string)  [unwired: 3 in]
      }
    }
    n103 = Wait (ms)(milliseconds to wait=w226) -> ()  [unwired: 1 out]
    n104 = Unbundle(w220) -> (w219:bool, "Unit Address (1)"=w217:u8, "VISA resource name out"=w216:refnum<visa-resource-name>, "error out"=w215:errorcluster)
    n105 = case shown="False" w250 {
      selector: w250 -> [w510 w517]
      tunnel: w253 -> [w509 w522]
      tunnel: w252 -> [w508 w521]
      tunnel: [w511 w520] -> w251
      tunnel: [w511 w519] -> w247
      tunnel: [w507 w516] -> w244
      frame False {
        w511 = "no QCM data"
        n106 = Bundle(w510, "VISA out"=w509, "error out"=w508) -> (w507:T11)  [unwired: 1 in]
      }
      frame True {
        # "SRS QCM"
        n107 = call "Elapsed Time2"() -> ("Elapsed Time (s)"=w523:dbl)  [unwired: 12 in, 7 out]
        n108 = call <instrlib>:"SrsQcm200FandR.vi"("VISA in"=w522, "Reference time in"=w523, "error in (no error)"=w521) -> ("VISA out"=w518:refnum<visa-resource-name>, "Frequency out"=w514:dbl, "Resistance out"=w513:dbl, "error out"=w512:errorcluster)  [unwired: 6 in, 3 out]
        "Freq (Hz)" <- w514
        "R (Ohm)" <- w513
        n109 = Number To Engineering String(4:w513) -> (0:w519:string)  [unwired: 3 in]
        n110 = Number To Engineering String(4:w514) -> (0:w520:string)  [unwired: 3 in]
        n111 = Bundle("Frequency out"=w514, "Resistance out"=w513) -> (→"Waveform Chart 7":T2)  [unwired: 1 in]
        n112 = Bundle(w517, "VISA out"=w518, "error out"=w512) -> (w516:T11)  [unwired: 1 in]
      }
    }
    n113 = case shown="False" w223 {
      selector: w223 -> [w494 w503]
      tunnel: w255 -> [w493 w497]
      tunnel: w254 -> [w492 w496]
      tunnel: [w491 w501] -> w245
      tunnel: ["no keithley 2420 data" w500] -> w246
      frame False {
        n114 = Bundle(w494, "VISA resource name out"=w493, "error out"=w492) -> (w491:T9)  [unwired: 1 in]
      }
      frame True {
        # "Keithley 2420"
        n115 = Wait (ms)(milliseconds to wait=u32 0) -> ()  [unwired: 1 out]
        n116 = call-poly <instrlib>:"Read.vi"("VISA resource name"=w497, "error in (no error)"=w496) -> ("VISA resource name out"=w504:refnum<visa-resource-name>, "Resistance"=w498:sgl, "error out"=w502:errorcluster)  [unwired: 7 in, 4 out]
        "Resistance (Ohm)" <- w498
        n117 = Bundle("Resistance"=w498) -> (→"Waveform Chart 4":cluster{"Resistance":sgl})  [unwired: 1 in]
        n118 = Number To Engineering String(4:w498) -> (0:w500:string)  [unwired: 3 in]
        n119 = Wait (ms)(milliseconds to wait=u32 200) -> ()  [unwired: 1 out]
        n120 = Bundle(w503, "VISA resource name out"=w504, "error out"=w502) -> (w501:T9)  [unwired: 1 in]
      }
    }
    n121 = case shown="True" w212 {
      selector: w212 -> [w269 w314]
      tunnel: w211 -> [w267 w316]
      tunnel: w213 -> [w268 w315]
      tunnel: [w268 w312] -> w210
      tunnel: [w267 w311] -> w209
      tunnel: [w269 w314] -> w208
      tunnel: w207 -> [w266 w289]
      tunnel: w206 -> [w265 w288]
      tunnel: [w266 w286] -> w205
      tunnel: [w265 w287] -> w204
      tunnel: [w264 refnum<visa-resource-name> refnum ("VISA resource name out")] -> w202
      tunnel: w203 -> [w264 _]
      tunnel: [w263 errorcluster {"status"=FALSE, "code"=0, "source"=""} ("error out")] -> w200
      tunnel: w201 -> [w263 _]
      frame False {
      }
      frame True {
        # "DAQ Pressure, Gas/Vapor Flows, & Butterfly Valve Control"
        # "Butterfly Valve"
        n122 = Wait (ms)(milliseconds to wait=u32 1000) -> ()  [unwired: 1 out]
        n123 = call-poly <vilib>:"DAQmx Read.vi"("task/channels in"=w315, "error in"=w316) -> ("task out"=w312:refnum<k21>, "data"=w303:dbl[], "error out"=w311:errorcluster)  [unwired: 11 in]
        "raw DVS DAQ data" <- w303
        n124 = Build Array("Set vapor flow (sccm)", "Set gas flow (sccm)") -> (w277:sgl[])
        n125 = Index Array(array=w303, index=4) -> (element=w299:dbl)
        n126 = Index Array(array=w303, index=0) -> (element=w291:dbl)
        "Vacuum Pressure (Torr)" <- w291
        "Waveform Chart 10" <- w291
        n127 = Index Array(array=w303, index=1) -> (element=w306:dbl)
        n128 = Index Array(array=w303, index=2) -> (element=w290:dbl)
        "Low pressure (Torr)" <- w290
        "Waveform Chart 9" <- w290
        n129 = Index Array(array=w303, index=3) -> (element=w301:dbl)
        n130 = Divide(x=w277, y=dbl[] [40.0, 40.0]) -> (x/y=w278:dbl[])
        n131 = Multiply(x=40.0, y=w299) -> (x*y=w283:dbl)
        n132 = Multiply(x=40.0, y=w301) -> (x*y=w280:dbl)
        n133 = Greater Or Equal?(x=w280, y=1.0) -> (x >= y?=w279:bool)
        n134 = Greater Or Equal?(x=w283, y=1.0) -> (x >= y?=w282:bool)
        n135 = call-poly <vilib>:"DAQmx Write.vi"("task/channels in"=w289, "data"=w278, "error in"=w288) -> ("task out"=w286:refnum<k21>, "error out"=w287:errorcluster)  [unwired: 10 in, 1 out]
        n136 = Multiply(x=100.0, y=w306) -> (x*y=w293:dbl)
        n137 = Select(t=w280, s=w279, f=0.0) -> (s? t:f=w272:dbl)
        "Gas flow (sccm)" <- w272
        n138 = Select(t=w283, s=w282, f=0.0) -> (s? t:f=w273:dbl)
        "Vapor flow (sccm)" <- w273
        n139 = Greater Than 0?(x=w293) -> (x > 0?=w296:bool)
        n140 = Select(t=w293, s=w296, f=0.0) -> (s? t:f=→"High pressure (Torr)" →"Waveform Chart 8":dbl)
        n141 = Bundle("f"=w272, "f"=w273) -> (→"Waveform Chart 2":cluster{"f":dbl, "f":dbl})  [unwired: 1 in]
        n142 = Bundle("Waveform"=w291, "Waveform"=w290) -> (→"Waveform Chart 11":cluster{"Waveform":dbl, "Waveform":dbl})  [unwired: 1 in]
      }
    }
    n143 = case shown="True" w219 {
      selector: w219 -> [_ w334]
      tunnel: [T9 {FALSE, "VISA resource name out"="", "error out"={"status"=FALSE, "code"=0, "source"=""}} w331] -> w218
      tunnel: w217 -> [_ w336]
      tunnel: w216 -> [_ w330]
      tunnel: w215 -> [_ w329]
      tunnel: ["no eurotherm data" w328] -> w214
      frame False {
      }
      frame True {
        w320 = u8 0 items=["Auto", "Manual"] ("Controller  Mode 2")
        w321 = u8 0 items=["None", "All", "Edit", "mod", "mAn", "Stby", "tmr"] ("Keylock 2")
        # "Eurotherm Temp Controller"
        n144 = Wait (ms)(milliseconds to wait=u32 100) -> ()  [unwired: 1 out]
        n145 = call <instrlib>:"Configure Keylock.vi"("VISA resource name"=w330, "Unit Address (1)"=w336, "Keylock"=w321, "error in (no error)"=w329) -> ("VISA resource name out"=w323:refnum<visa-resource-name>, "error out"=w322:errorcluster)  [unwired: 10 in]
        n146 = call <instrlib>:"Controller Mode.vi"("VISA resource name"=w323, "Unit Address (1)"=w336, "Controller Mode (0: Auto)"=w320, "error in (no error)"=w322) -> ("VISA resource name out"=w338:refnum<visa-resource-name>, "error out"=w341:errorcluster)  [unwired: 10 in]
        n147 = call <instrlib>:"Configure Setpoint.vi"("VISA resource name"=w338, "Unit Address (1)"=w336, "Setpoint Value (0)"="Setpoint (C)", "error in (no error)"=w341) -> ("VISA resource name out"=w339:refnum<visa-resource-name>, "error out"=w340:errorcluster)  [unwired: 10 in]
        n148 = call <instrlib>:"Read Process Variables.vi"("VISA resource name"=w339, "Unit Address (1)"=w336, "error in (no error)"=w340) -> ("VISA resource name out"=w325:refnum<visa-resource-name>, "Process Value"=w327:sgl, "error out"=w324:errorcluster)  [unwired: 9 in, 1 out]
        "Temp (C)" <- w327
        n149 = Bundle("Process Value"=w327, "Setpoint (C)"="Setpoint (C)") -> (→"Temp":cluster{"Process Value":sgl, "Setpoint (C)":sgl})  [unwired: 1 in]
        n150 = call <instrlib>:"Error Message.vi"("VISA resource name"=w325, "error in (no error)"=w324) -> ("VISA resource name out"=w333:refnum<visa-resource-name>, "error out"=w332:errorcluster)  [unwired: 9 in, 3 out]
        n151 = Number To Engineering String(2:i16 5 ("width (-)"), 4:w327) -> (0:w328:string)  [unwired: 2 in]
        n152 = Bundle(w334, "VISA resource name out"=w333, "error out"=w332) -> (w331:T9)  [unwired: 1 in]
      }
    }
    n153 = call "Elapsed Time"() -> ("Elapsed Time (s)"=w236:dbl)  [unwired: 12 in, 7 out]
    n154 = Divide(x=w236, y=60.0) -> (x/y=w222:dbl)
    "Elapsed (min)" <- w222
    n155 = Number To Engineering String(4:w222) -> (0:w261:string)  [unwired: 3 in]
    n156 = case shown="False" "Auto stop?" {
      tunnel: w222 -> [_ w378]
      tunnel: [FALSE w380] -> w233
      frame False {
      }
      frame True {
        n157 = Greater Or Equal?(x=w378, y="Stop after (min)") -> (x >= y?=w380:bool)
        n158 = Subtract(x="Stop after (min)", y=w378) -> (x-y=→"min remaining":dbl)
      }
    }
    n159 = Get Date/Time In Seconds() -> (seconds since 1Jan1904=w262:timestamp)
    n160 = Or(x=w233, y="stop") -> (x .or. y?=w237:bool)
    n161 = Format Date/Time String(seconds (now)=w262) -> (date/time string=w256:string)  [unwired: 2 in]
    n162 = Build Array(w256, w261, w240, w246, w251, w247, w248, w228, w214, "DATA COMMENTS") -> (w257:string[])
  }
  n163 = Unbundle(w51) -> (w50:bool, "VISA resource name out"=w49:refnum<visa-resource-name>, "error out"=w48:errorcluster)
  n164 = Unbundle(w57) -> (w56:bool, "VISA out"=w55:refnum<visa-resource-name>, "error out"=w54:errorcluster)
  n165 = Unbundle(w61) -> (w60:bool, "VISA resource name out"=w59:refnum<visa-resource-name>, "error out"=w58:errorcluster)
  n166 = Get Date/Time In Seconds() -> (seconds since 1Jan1904=w75:timestamp)
  n167 = case shown="True" w60 {
    tunnel: w59 -> [_ w554]
    tunnel: w58 -> [w551 w553]
    tunnel: [w551 w552] -> w62
    frame False {
    }
    frame True {
      n168 = call <instrlib>:"Enable Output.vi"("error in (no error)"=w553, "Enable Output (T: Enable)"=FALSE, "VISA resource name"=w554) -> ("error out"=w555:errorcluster, "VISA resource name out"=w557:refnum<visa-resource-name>)  [unwired: 7 in]
      n169 = call <instrlib>:"Close.vi"("error in (no error)"=w555, "VISA resource name"=w557) -> ("error out"=w552:errorcluster)  [unwired: 9 in]
    }
  }
  n170 = case shown="True" w56 {
    tunnel: w54 -> [w558 w561]
    tunnel: [w558 w560] -> w63
    tunnel: w55 -> [_ w559]
    frame False {
    }
    frame True {
      n171 = call <instrlib>:"srsQcm200Close.vi"("error in"=w561, "Visa in"=w559) -> ("error out"=w560:errorcluster)  [unwired: 3 in]
    }
  }
  n172 = Unbundle(w25) -> (w24:bool, "VISA resource name out"=w23:refnum<visa-resource-name>, "error out"=w22:errorcluster)
  n173 = Format Date/Time String(seconds (now)=w75) -> (date/time string=→"Starting time":string)  [unwired: 2 in]
  n174 = case shown="True" w14 {
    tunnel: [w562 w576] -> w7
    tunnel: w16 -> [_ w575]
    tunnel: w15 -> [_ w574]
    tunnel: w9 -> [_ w570]
    tunnel: w8 -> [_ w569]
    tunnel: [w562 w568] -> w6
    tunnel: [w562 w565] -> w1
    tunnel: w3 -> [_ w564]
    tunnel: w2 -> [_ w563]
    frame False {
      w562 = errorcluster {"status"=FALSE, "code"=0, "source"=""} ("error out")
    }
    frame True {
      n175 = call <vilib>:"DAQmx Stop Task.vi"("task/channels in"=w570, "error in"=w569) -> ("task out"=w572:refnum<k21>, "error out"=w571:errorcluster)  [unwired: 12 in]
      n176 = call <vilib>:"DAQmx Stop Task.vi"("task/channels in"=w575, "error in"=w574) -> ("task out"=w573:refnum<k21>, "error out"=w577:errorcluster)  [unwired: 12 in]
      n177 = VISA Clear(VISA resource name=w564, error in (no error)=w563) -> (VISA resource name out=w567:refnum<visa-resource-name>, error out=w566:errorcluster)
      n178 = call <vilib>:"DAQmx Clear Task.vi"("task in"=w572, "error in"=w571) -> ("error out"=w568:errorcluster)  [unwired: 13 in]
      n179 = call <vilib>:"DAQmx Clear Task.vi"("task in"=w573, "error in"=w577) -> ("error out"=w576:errorcluster)  [unwired: 13 in]
      n180 = VISA Close(VISA resource name=w567, error in (no error)=w566) -> (error out=w565:errorcluster)
    }
  }
  n181 = case shown="True" w50 {
    tunnel: w49 -> [_ w581]
    tunnel: w48 -> [w578 w580]
    tunnel: [w578 w579] -> w47
    frame False {
    }
    frame True {
      n182 = VISA Close(VISA resource name=w581, error in (no error)=w580) -> (error out=w579:errorcluster)
    }
  }
  n183 = case shown="True" w24 {
    tunnel: w23 -> [_ w585]
    tunnel: w22 -> [_ w584]
    tunnel: [errorcluster {"status"=FALSE, "code"=0, "source"=""} ("error out") w583] -> w12
    frame False {
    }
    frame True {
      n184 = call <instrlib>:"Close.vi"("VISA resource name"=w585, "error in (no error)"=w584) -> ("error out"=w583:errorcluster)  [unwired: 13 in]
    }
  }
  n185 = Merge Errors(w12, w6, w7, w1) -> (w13:errorcluster)
  n186 = Merge Errors(w47, w62, w63, w30, w13) -> (w73:errorcluster)
  n187 = call <vilib>:"Simple Error Handler.vi"("error in (no error)"=w73) -> ("error out"=→"ERRORS":errorcluster)  [unwired: 4 in, 4 out]
  n188 = Build Array("date/time", "min elapsed", "J-KEM temp (C)", "Keithley 2420 resistance (Ohm)" ("element"), "QCM freq (Hz)", "QCM resistance (Ohm)", "O2 partial pressure (Torr)" ("element"), "O2 concentration (PPM)" ("element"), "eurotherm temp (C)" ("element"), "user comment" ("element")) -> (w38:string[])
  n189 = call-poly <vilib>:"Write To Spreadsheet File.vi"("1D data"=w38, "file path (dialog if empty)"=w29) -> ("new file path (Not A Path if cancelled)"=w39:path)  [unwired: 6 in]
  n190 = call-poly <vilib>:"Write To Spreadsheet File.vi"("append to file? (new file:F)"=TRUE, "2D data"=w72, "file path (dialog if empty)"=w39) -> ()  [unwired: 5 in, 1 out]
